vi "Uninit.vi"(2 "Container State":T1, 3 "Display State":T2) -> ()   [LabVIEW 2018, in "Hide Panel.xctl"]
uses:
  Hide Panel.xctl
  State.ctl
  <vilib>/_xctls/Container State.ctl
  <vilib>/_xctls/XControlSupport.lvlib
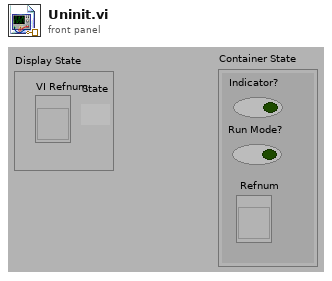
[diagram p1: front panel]
types:
  T1 = typedef "XControlSupport.lvlib/Container State.ctl" = cluster{"Indicator?":bool, "Run Mode?":bool, " Refnum":refnum<vi>}
  T2 = typedef "Hide Panel.xctl/State.ctl" = cluster{"VI Refnum":refnum<vi>, "State":bool}
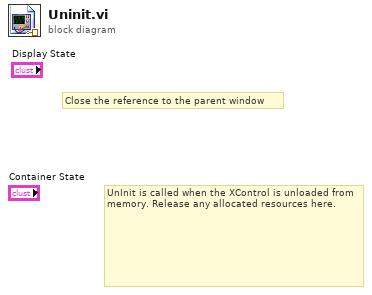
[diagram p0: block diagram]
diagram:
  # "Close the reference to the parent window"
  # "UnInit is called when the XControl is unloaded from memory. Release any allocated resources here."
